vi "Camera.getBuffer.vi"(8 "error in (no error)":errorcluster, 10 "Get Image (-1: latest)":i32=-1, 11 "Camera.Simulated in":refnum<class "Camera.IMAQdx.lvclass">) -> (0 "error out":errorcluster, 2 "pixmap":u32[][](array[numeric]), 3 "Camera.Simulated out":refnum<class "Camera.IMAQdx.lvclass">)   [LabVIEW 2020, in "Camera.IMAQdx.lvclass"]
uses:
  Camera.IMAQdx.lvclass
  Camera.IMAQdx.lvclass/Camera.IMAQdx.ctl
  <vilib>/vision/driver/NI_Vision_Acquisition_Software.lvlib
  <vilib>/vision/driver/IMAQdx.llb/IMAQdx Buffer Number Mode.ctl
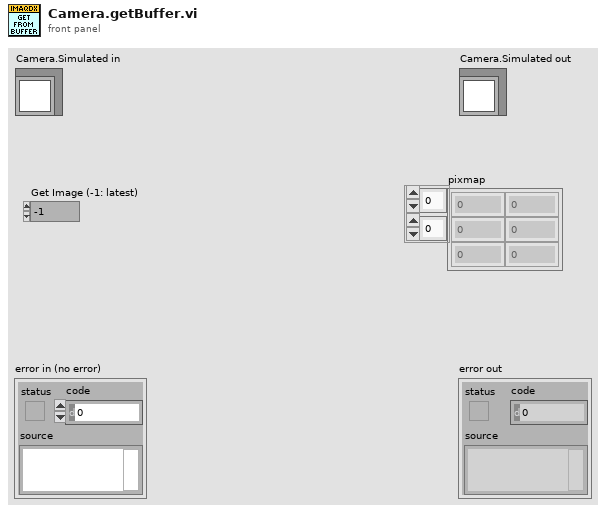
[diagram p1: front panel]
types:
  T1 = typedef "NI_Vision_Acquisition_Software.lvlib/IMAQdx Buffer Number Mode.ctl" = enum32{"Next", "Last", "Buffer Number", "Every", "Last New"}
  T2 = typedef "IMAQ Image.ctl" = refnum<image>
  T3 = typedef "IMAQdx.ctl" = refnum<k21>
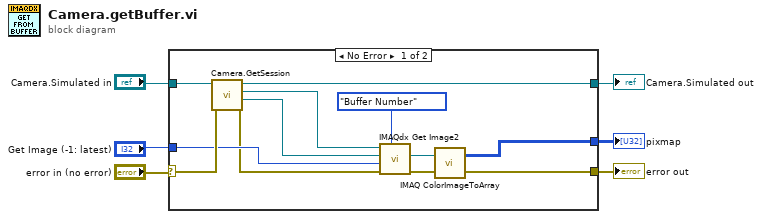
[diagram p0: block diagram]
diagram:
  n1 = case shown="No Error" "error in (no error)" {
    selector: "error in (no error)" -> [w17 w20]
    tunnel: [w8 w20] -> w2
    tunnel: [w16 w19] -> w1
    tunnel: "Camera.Simulated in" -> [w18 w19]
    tunnel: "Get Image (-1: latest)" -> [w14 _]
    tunnel: [w7 _] -> w3
    frame No Error {
      n2 = call "Camera.GetSession.vi"("error in (no error)"=w17, "Camera.Simulated"=w18) -> ("error out"=w12:errorcluster, "Image"=w11:T2, "Session"=w15:T3, "Camera.Simulated"=w16:refnum<class "Camera.IMAQdx.lvclass">)  [unwired: 6 in]
      n3 = call <vilib>:"IMAQdx Get Image2.vi"("Buffer Number Mode (Next)"=IMAQdx_Buffer_Number_Mode."Buffer Number", "error in"=w12, "Buffer Number In"=w14, "Image In"=w11, "Session In"=w15) -> ("error out"=w9:errorcluster, "Image Out"=w10:T2)  [unwired: 3 in, 2 out]
      n4 = call "IMAQ ColorImageToArray"("Image"=w10, "error in (no error)"=w9) -> ("Image Pixels (U32)"=w7:u32[][], "error out"=w8:errorcluster)  [unwired: 2 in, 1 out]
    }
    frame Error {
    }
  }
  "error out" <- w2
  "Camera.Simulated out" <- w1
  "pixmap" <- w3
